vi "一线双色计算.vi"(1 "输入一维数组":dbl[](array[numeric]), 2 "right corsor":dbl=5.0, 3 "left corsor":dbl=5.0) -> (0 "输出波形数组":dbl[][](array[numeric]))   [LabVIEW 2014]
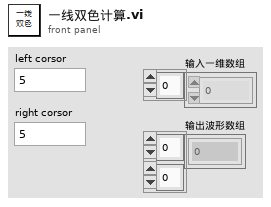
[diagram p1: front panel]
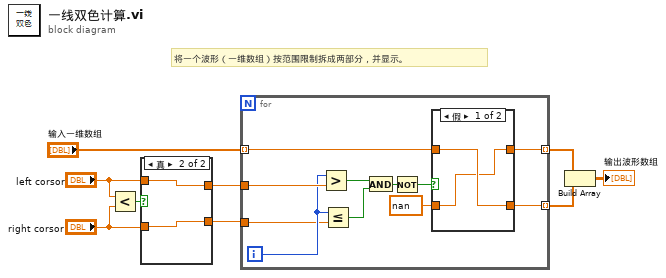
[diagram p0: block diagram]
diagram:
  # "将一个波形（一维数组）按范围限制拆成两部分，并显示。"
  n1 = Less?(x="left corsor", y="right corsor") -> (x < y?=w5:bool)
  n2 = case shown="真" w5 {
    tunnel: "left corsor" -> [w11 w13]
    tunnel: [w10 w13] -> w3
    tunnel: "right corsor" -> [w10 w12]
    tunnel: [w11 w12] -> w1
    frame False {
    }
    frame True {
    }
  }
  n3 = for {
    tunnel: w3 -> [w24]
    tunnel: "输入一维数组" -> [w23] mode=indexing
    tunnel: [w21] -> w6 mode=indexing
    tunnel: [w20] -> w7 mode=indexing
    tunnel: w1 -> [w18]
    i -> [w19]
    n4 = Greater?(x=w19, y=w24) -> (0:w16:bool)
    n5 = Less Or Equal?(x=w19, y=w18) -> (x <= y?=w15:bool)
    n6 = And(x=w16, y=w15) -> (x .and. y?=w17:bool)
    n7 = Not(x=w17) -> (.not. x?=w14:bool)
    n8 = case shown="假" w14 {
      tunnel: w23 -> [w26 w28]
      tunnel: nan -> [w25 w27]
      tunnel: [w25 w28] -> w21
      tunnel: [w26 w27] -> w20
      frame False {
      }
      frame True {
      }
    }
  }
  n9 = Build Array(w6, w7) -> (→"输出波形数组":dbl[][])
